vi "Helper Stop Core.vi"(8 "error in (no error)":errorcluster, 11 "Analog Reader Helper in":refnum<class "Analog Reader Helper.lvclass">) -> (0 "error out":errorcluster, 3 "Analog Reader Helper out":refnum<class "Analog Reader Helper.lvclass">)   [LabVIEW 2024, in "DAQmx Actor.lvlib" / "Analog Reader Helper.lvclass"]
uses:
  Analog Reader Helper.lvclass
  Analog Reader Helper.lvclass/Analog Reader Helper.ctl
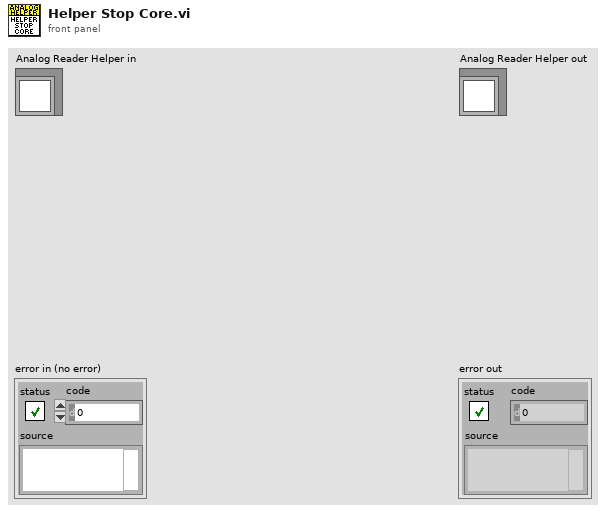
[diagram p1: front panel]
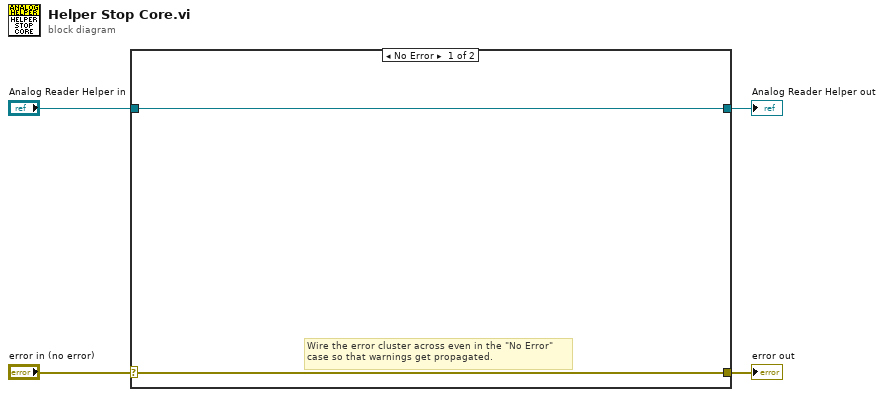
[diagram p0: block diagram]
diagram:
  n1 = case shown="No Error" "error in (no error)" {
    selector: "error in (no error)" -> [w5 w8]
    tunnel: [w5 w8] -> w3
    tunnel: [w6 w7] -> w1
    tunnel: "Analog Reader Helper in" -> [w6 w7]
    frame No Error {
      # "Wire the error cluster across even in the \"No Error\"\ncase so that warnings get propagated."
    }
    frame Error {
    }
  }
  "error out" <- w3
  "Analog Reader Helper out" <- w1
